vi "Xtimer.vi"(9 "Reset":bool) -> (1 "Time (sec)":dbl)   [LabVIEW 2020]
panel:
  in  "stop":bool
  # "TIIMER"
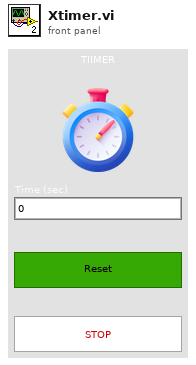
[diagram p1: front panel]
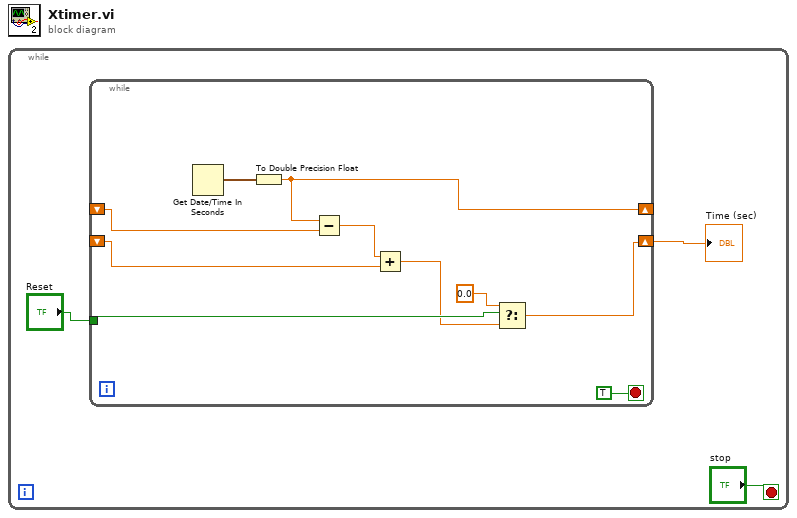
[diagram p0: block diagram]
diagram:
  n1 = while {
    stop <- "stop" stop-if-true
    n2 = while {
      shift-right: [w12] -> _
      shift-left: _ -> [w11]
      shift-right: [w6] -> w3
      shift-left: _ -> [w9]
      tunnel: "Reset" -> [w8]
      stop <- TRUE stop-if-true
      n3 = Get Date/Time In Seconds() -> (seconds since 1Jan1904=w13:timestamp)
      n4 = To Double Precision Float(number=w13) -> (double precision float=w12:dbl)
      n5 = Subtract(x=w12, y=w11) -> (x-y=w10:dbl)
      n6 = Add(x=w10, y=w9) -> (x+y=w7:dbl)
      n7 = Select(t=0.0, s=w8, f=w7) -> (s? t:f=w6:dbl)
    }
    "Time (sec)" <- w3
  }
